vi "总磷总氮流程质控自动启动.vi"(9 "总磷量程切换":enum32{"H", "L", "AUTO"}(ring)=enum."AUTO", 10 "总氮量程切换":enum32{"H", "L", "AUTO"}(ring)=enum."AUTO", 11 "参数":T1={"是否启用仪器"=FALSE, "CODMn"={"启动测量模式"={"测量模式"=enum."水样测量"}, "确定按钮"=TRUE}, "启动模块"={"氨氮"=FALSE, "总磷"=FALSE, "总氮"=FALSE, "COD"=FALSE}, "常规启动"=FALSE, "直接启动"=FALSE}) -> ()   [LabVIEW 2016, in "质控单元.lvlib"]
uses:
  PLC/PLC.lvlib
panel:
  out "枚举 2":enum16{"初始化", "采配水启动", "等待", "配水", "排水", "结束"}(ring)
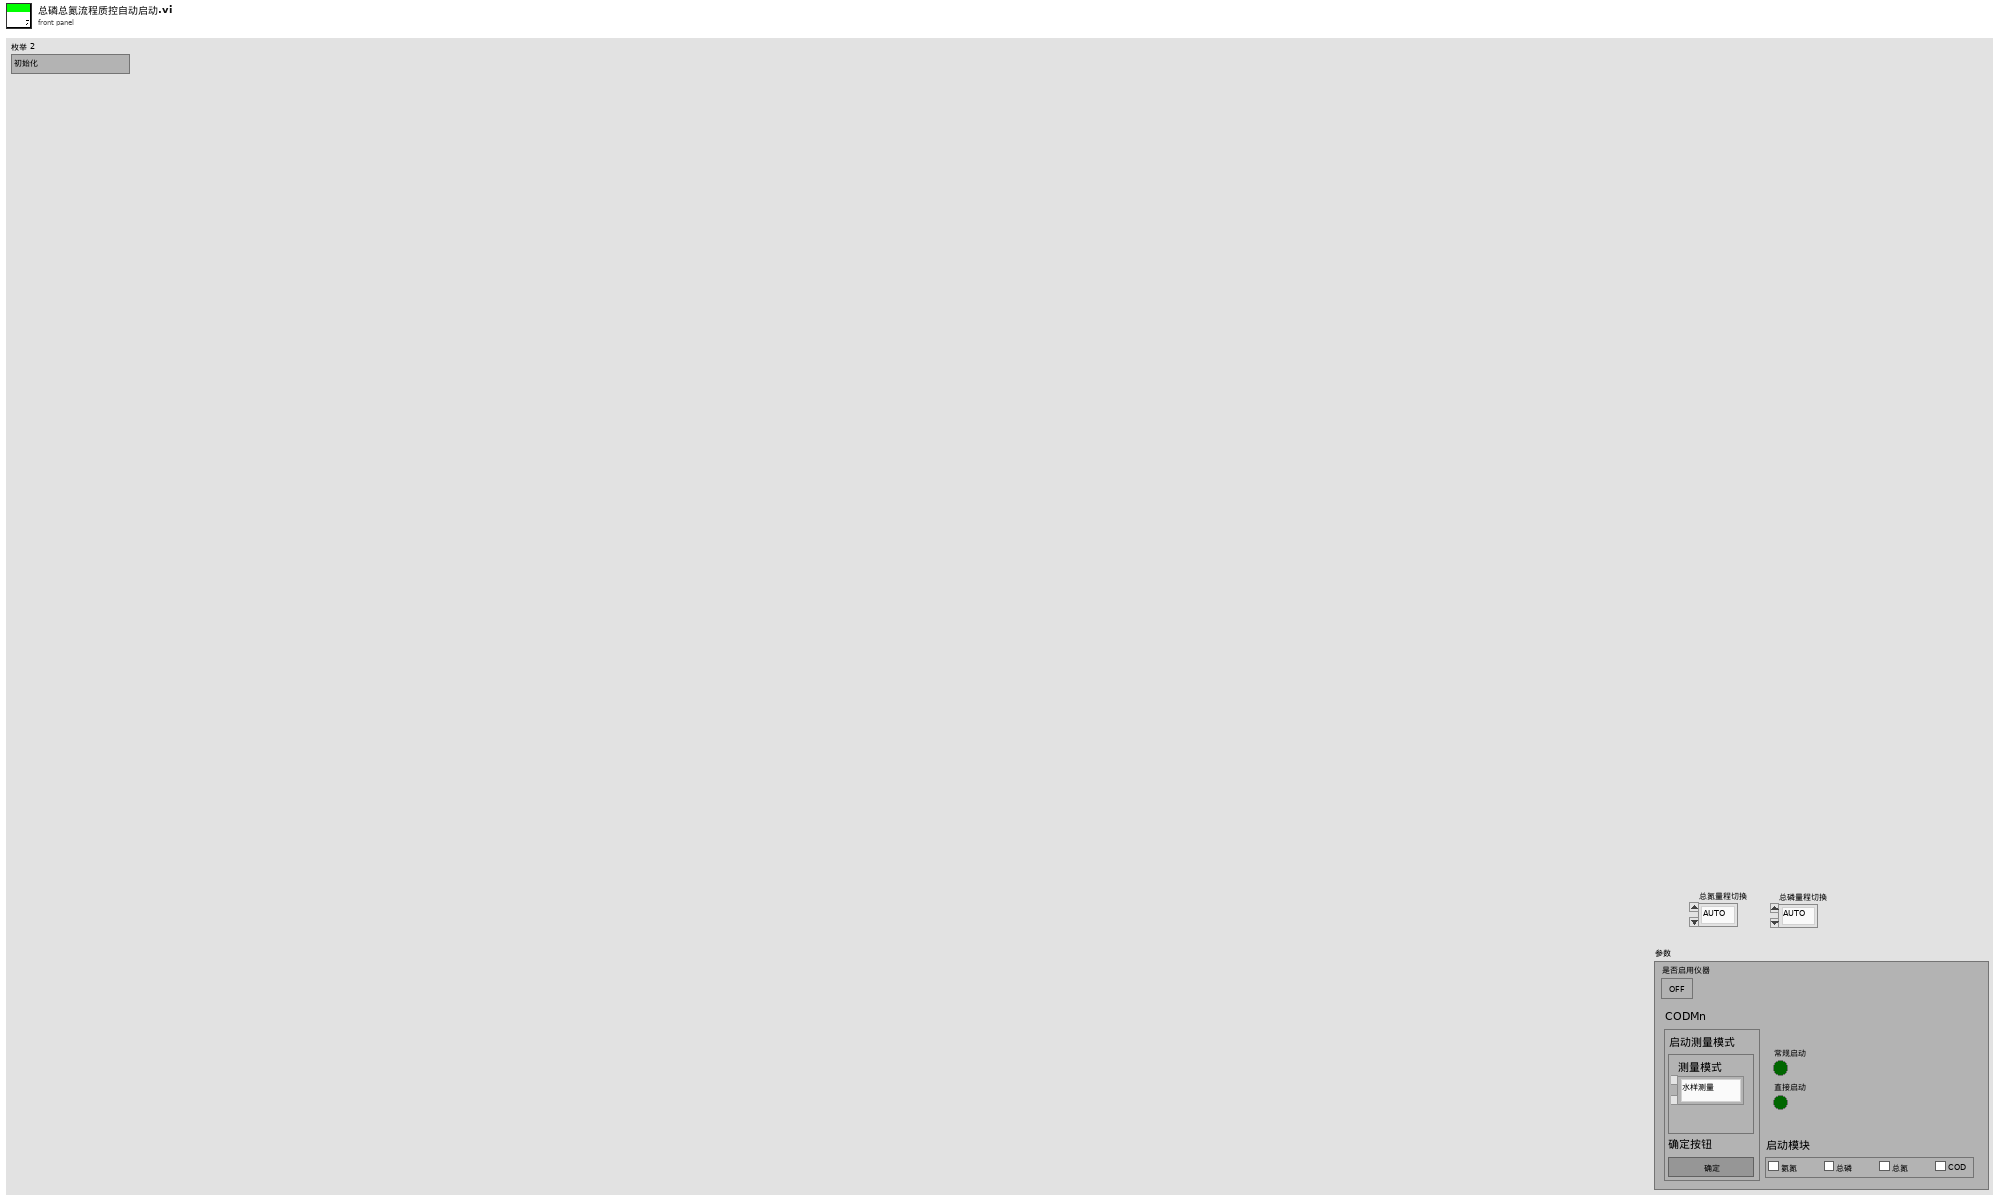
[diagram p1: front panel]
types:
  T1 = cluster{"是否启用仪器":bool, "CODMn":cluster{"启动测量模式":cluster{"测量模式":enum16{"水样测量", "标样核查", "加标回收", "平行样", "校零", "校标"}}, "确定按钮":bool}, "启动模块":cluster{"氨氮":bool, "总磷":bool, "总氮":bool, "COD":bool}, "常规启动":bool, "直接启动":bool}
  T2 = cluster{"R0":i16, "R1":i16, "R2":i16, "R3":i16, "R4":i16, "R5":i16, "R6":i16, "R7":i16, "R8":i16, "R9":i16, "R10":i16, "R11":i16, "R12":i16, "R13":i16, "R14":i16, "R15":i16, "R16":i16, "R17":i16, "R18":i16, "R19":i16, "R20":i16, "R21":i16, "R22":i16, "R23":i16, "R24":i16, "R25":i16, "R26":i16, "R27":i16, "R28":i16, "R29":i16, "R30":i16, "R31":i16, "R32":i16, "R33":i16, "R34":i16, "R35":i16, "R36":i16, "R37":i16, "R38":i16, "R39":i16, "R40":i16, "R41":i16, "R42":i16, "R43":i16, "R44":i16, "R45":i16, "R46":i16, "R47":i16, "R48":i16, "R49":i16, "R50":i16, "R51":i16, "R52":i16, "R53":i16, "R54":i16, "R55":i16, "R56":i16}
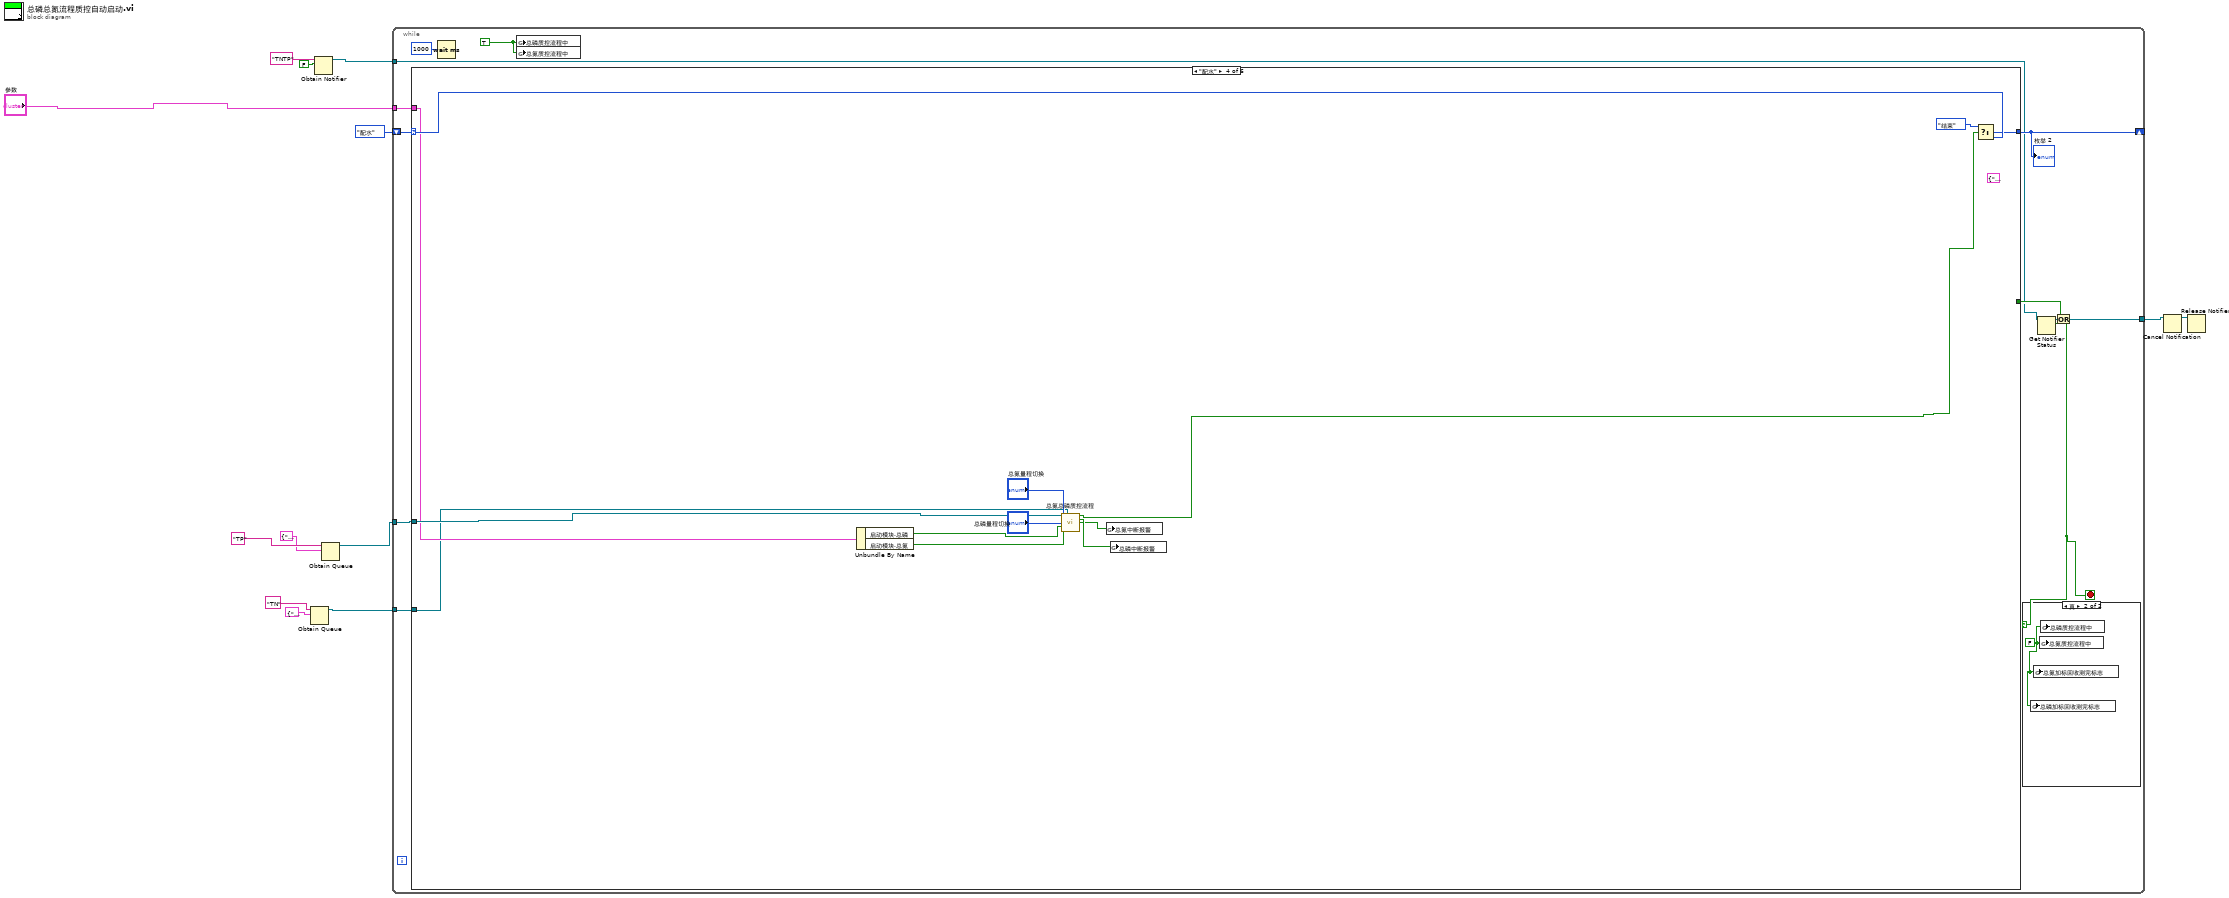
[diagram p0: block diagram]
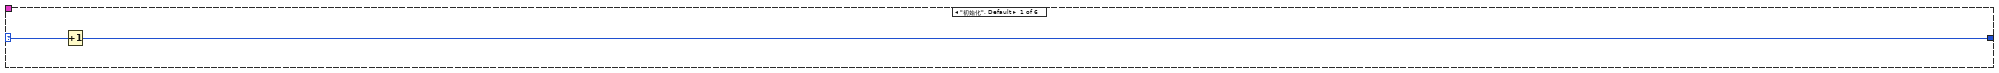
[diagram p3: hidden frame]
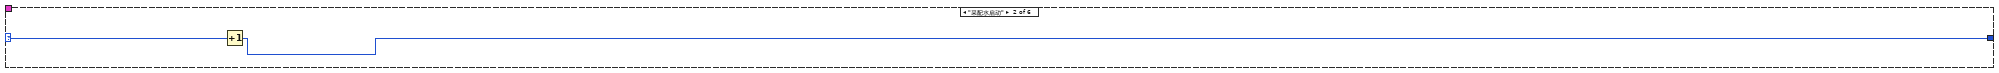
[diagram p4: hidden frame]
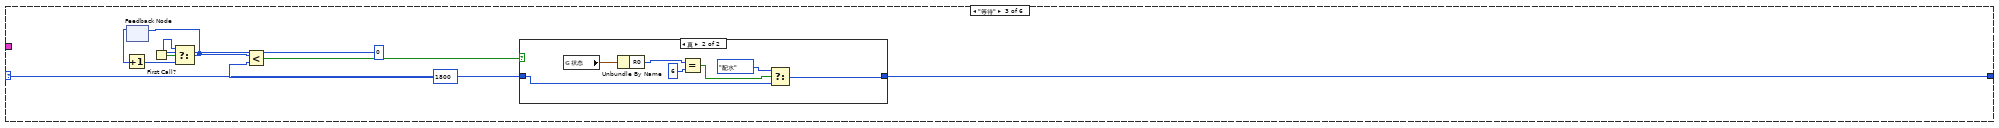
[diagram p5: hidden frame]
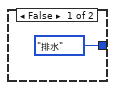
[diagram p6: hidden frame]
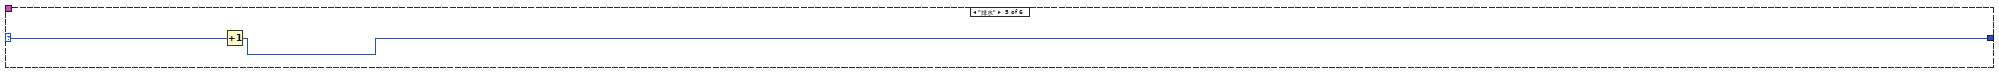
[diagram p7: hidden frame]
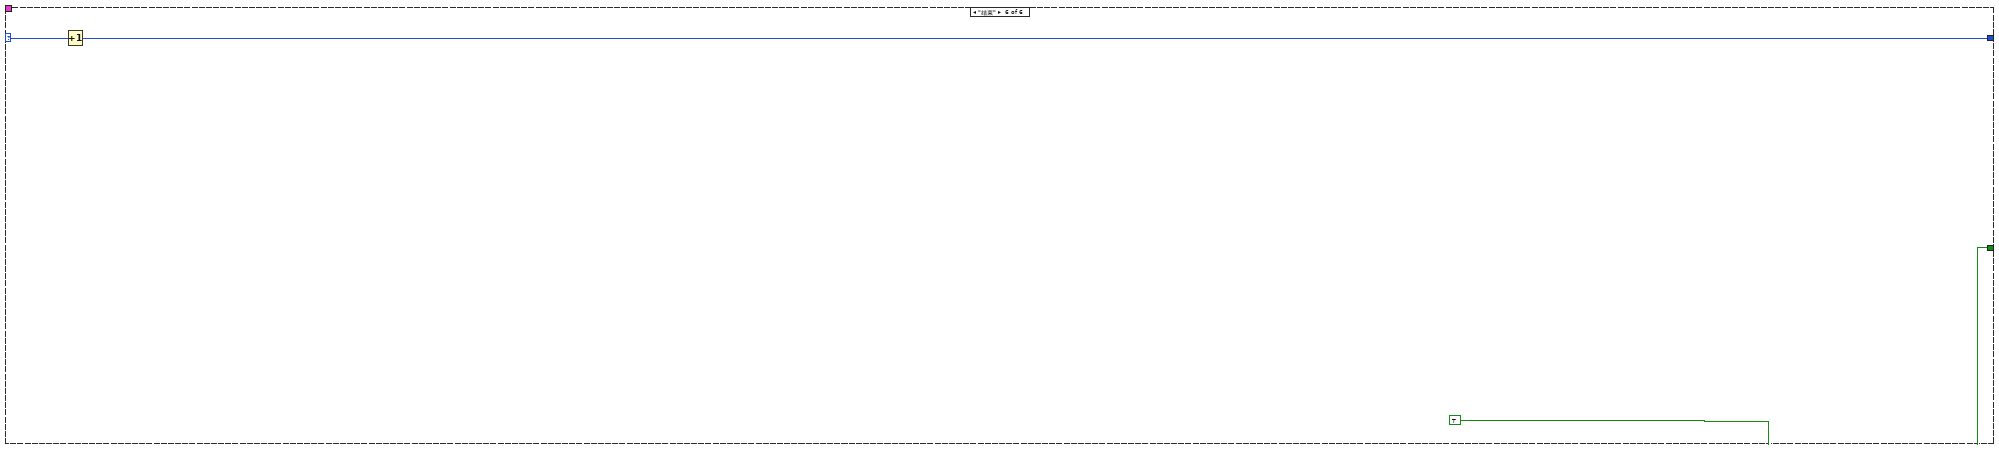
[diagram p8: hidden frame]
diagram:
  n1 = Obtain Queue(name (unnamed)="TN" ("名称（未命名）"), element data type=cluster{"命令":string, "data":variant} {"命令"="", "data"=variant}) -> (queue out=w1:refnum<queue>)  [unwired: 3 in, 2 out]
  n2 = Obtain Notifier(name (unnamed)="TNTP" ("名称（未命名）"), notification data type=FALSE) -> (notifier out=w6:refnum<notifier>)  [unwired: 2 in, 2 out]
  n3 = Obtain Queue(name (unnamed)="TP" ("名称（未命名）"), element data type=cluster{"命令":string, "data":variant} {"命令"="", "data"=variant}) -> (queue out=w9:refnum<queue>)  [unwired: 3 in, 2 out]
  n4 = while {
    shift-right: [w24] -> _
    shift-left: enum16{"初始化", "采配水启动", "等待", "配水", "排水", "结束"}."配水" ("枚举") -> [w25]
    tunnel: w9 -> [w22]
    tunnel: "参数" -> [w21]
    tunnel: w6 -> [w18]
    tunnel: [w17] -> w4
    tunnel: w1 -> [w14]
    stop <- w15 stop-if-true
    w16 = TRUE ("总磷质控流程中")
    n5 = case shown="\"配水\"" w25 {
      selector: w25 -> [w28 w30 w37 w59 w62 w65]
      tunnel: [w27 w29 w36 w58 w61 w64] -> w24
      tunnel: [_ _ _ _ _ TRUE] -> w20
      tunnel: w22 -> [_ _ _ w57 _ _]
      tunnel: w21 -> [_ _ _ w51 _ _]
      tunnel: w14 -> [_ _ _ w48 _ _]
      frame "初始化", Default {
        n6 = Increment(x=w28) -> (x+1=w27:enum16{"初始化", "采配水启动", "等待", "配水", "排水", "结束"})
      }
      frame "采配水启动" {
        n7 = Increment(x=w30) -> (x+1=w29:enum16{"初始化", "采配水启动", "等待", "配水", "排水", "结束"})
      }
      frame "等待" {
        n8 = feedback #1() -> (w33:i32)  [unwired: 1 in]
        n9 = Increment(x=w33) -> (x+1=w32:i32)
        n10 = First Call?() -> (First Call?: T/F=w34:bool)
        n11 = Select(t=0, s=w34, f=w32) -> (s? t:f=w31:i32)
        n12 = feedback-in #1(w31) -> ()
        n13 = Less?(x=w31, y=1800) -> (x < y?=w38:bool)
        n14 = case shown="真" w38 {
          tunnel: w37 -> [_ w42]
          tunnel: [enum16{"初始化", "采配水启动", "等待", "配水", "排水", "结束"}."排水" ("枚举") w41] -> w36
          frame False {
          }
          frame True {
            n15 = global read "采配水全局变量.vi" "状态"() -> (w47:T2)
            n16 = Unbundle By Name(w47) -> ("R0"=w46:i16)
            n17 = Equal?(x=w46, y=i16 6) -> (x = y?=w44:bool)
            n18 = Select(t=enum16{"初始化", "采配水启动", "等待", "配水", "排水", "结束"}."配水" ("枚举"), s=w44, f=w42) -> (s? t:f=w41:enum16{"初始化", "采配水启动", "等待", "配水", "排水", "结束"})
          }
        }
      }
      frame "配水" {
        (unwired) cluster{"命令":string, "data":variant} {"命令"="启动", "data"=variant(cluster{"站号":u16, "控制命令输出":u16[]} {"站号"=1, "控制命令输出"=[256, 0]})} ("元素")
        n19 = Unbundle By Name(w51) -> ("启动模块.总磷"=w50:bool, "启动模块.总氮"=w49:bool)
        n20 = call "总氮总磷质控流程.vi"("队列输入TP"=w57, "队列输入TN"=w48, "总氮量程切换"="总氮量程切换", "总磷量程切换"="总磷量程切换", "总磷"=w50, "总氮"=w49) -> ("布尔"=w54:bool, "总磷中断报警"=w53:bool, "总氮中断报警"=w52:bool)  [unwired: 7 in]
        n21 = global write "质控中断报警全局.vi" "总氮中断报警"(w52) -> ()
        n22 = global write "质控中断报警全局.vi" "总磷中断报警"(w53) -> ()
        n23 = Select(t=enum16{"初始化", "采配水启动", "等待", "配水", "排水", "结束"}."结束" ("枚举"), s=w54, f=w59) -> (s? t:f=w58:enum16{"初始化", "采配水启动", "等待", "配水", "排水", "结束"})
      }
      frame "排水" {
        n24 = Increment(x=w62) -> (x+1=w61:enum16{"初始化", "采配水启动", "等待", "配水", "排水", "结束"})
      }
      frame "结束" {
        n25 = Increment(x=w65) -> (x+1=w64:enum16{"初始化", "采配水启动", "等待", "配水", "排水", "结束"})
      }
    }
    "枚举 2" <- w24
    n26 = Wait (ms)(milliseconds to wait=u32 1000 ("等待时间（毫秒）")) -> ()  [unwired: 1 out]
    n27 = global write "质控测完标志全局 1.vi" "总磷质控流程中"(w16) -> ()
    n28 = global write "质控测完标志全局 1.vi" "总氮质控流程中"(w16) -> ()
    n29 = Get Notifier Status(notifier=w18) -> (notifier out=w17:refnum<notifier>, current notification=w19:bool)  [unwired: 1 in, 3 out]
    n30 = Or(x=w20, y=w19) -> (x .or. y?=w15:bool)
    n31 = case shown="真" w15 {
      frame False {
      }
      frame True {
        w26 = FALSE ("总氮质控流程中")
        n32 = global write "质控测完标志全局 1.vi" "总磷加标回收测完标志"(w26) -> ()
        n33 = global write "质控测完标志全局 1.vi" "总氮加标回收测完标志"(w26) -> ()
        n34 = global write "质控测完标志全局 1.vi" "总氮质控流程中"(w26) -> ()
        n35 = global write "质控测完标志全局 1.vi" "总磷质控流程中"(w26) -> ()
      }
    }
  }
  n36 = Cancel Notification(0:w4) -> (8:w5:refnum<notifier>)  [unwired: 1 in, 2 out]
  n37 = Release Notifier(notifier=w5) -> ()  [unwired: 2 in, 3 out]
